vi "ws_www template header.vi"(8 "error in (no error)":errorcluster, 11 "Template Content (\"\")":string) -> (0 "error out":errorcluster, 3 "Template Content":string)   [LabVIEW 2011]
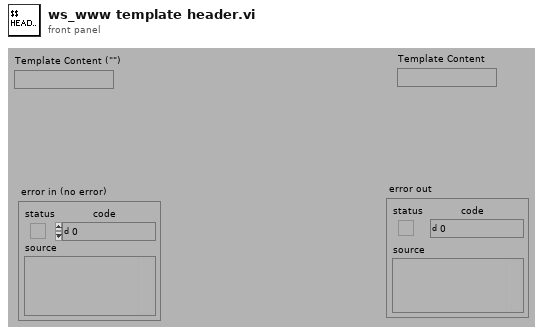
[diagram p1: front panel]
types:
  T1 = typedef "Keyed Array.ctl" = cluster{"keys":string[], "values":string[]}
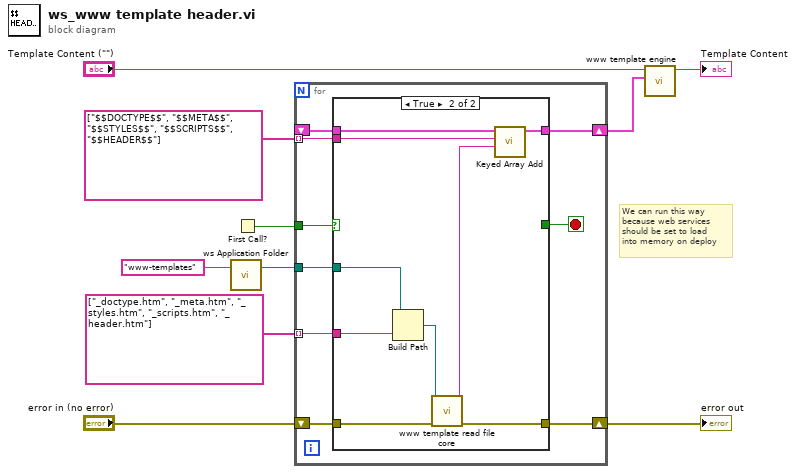
[diagram p0: block diagram]
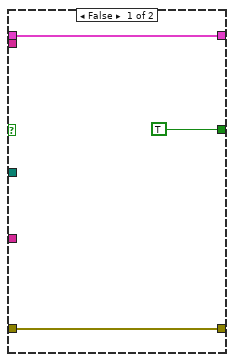
[diagram p2: hidden frame]
diagram:
  # "We can run this way\nbecause web services\nshould be set to load\ninto memory on deploy"
  n1 = call "ws Application Folder.vi"("Relative Path (\"\" - Folder)"="www-templates" ("name or relative path")) -> ("Application Folder"=w2:path)  [unwired: 2 in]
  n2 = First Call?() -> (First Call?: T/F=w1:bool)
  n3 = for {
    tunnel: w2 -> [w19]
    tunnel: string[] ["_doctype.htm", "_meta.htm", "_styles.htm", "_scripts.htm", "_header.htm"] -> [w18] mode=indexing
    shift-right: [w16] -> w5
    shift-left: "error in (no error)" -> [w17]
    shift-right: [w15] -> w7
    shift-left: _ -> [w14]
    tunnel: string[] ["$$DOCTYPE$$", "$$META$$", "$$STYLES$$", "$$SCRIPTS$$", "$$HEADER$$"] -> [w13] mode=indexing
    tunnel: w1 -> [w12]
    stop <- w11 stop-if-true
    n4 = case shown="True" w12 {
      tunnel: w19 -> [_ w31]
      tunnel: w18 -> [_ w30]
      tunnel: w17 -> [w21 w28]
      tunnel: [w21 w27] -> w16
      tunnel: [w22 w26] -> w15
      tunnel: w14 -> [w22 w25]
      tunnel: w13 -> [_ w24]
      tunnel: [TRUE _] -> w11
      frame False {
      }
      frame True {
        n5 = Build Path(base path=w31, name or relative path=w30) -> (appended path=w29:path)
        n6 = call "www template read file core.vi"("error in (no error)"=w28, "Path"=w29) -> ("error out"=w27:errorcluster, "File Content"=w23:string)  [unwired: 8 out]
        n7 = call <vilib>:"Keyed Array Add.vi"("value"=w23, "key"=w24, "array in"=w25) -> ("array out"=w26:T1)  [unwired: 2 in, 2 out]
      }
    }
  }
  "error out" <- w5
  n8 = call "www template engine.vi"("Template Dictionary (empty)"=w7, "Template String (\"\")"="Template Content (\"\")") -> ("Template String out"=→"Template Content":string)  [unwired: 1 in, 8 out]
